vi "test Connector Pane.vi"(8 "error in (no error)":errorcluster, 11 "TestCase in":refnum<class "Embedded Data Logger Unit Tests.lvclass">) -> (0 "error out":errorcluster, 3 "TestCase out":refnum<class "Embedded Data Logger Unit Tests.lvclass">)   [LabVIEW 2027, in "Embedded Data Logger Unit Tests.lvclass"]
uses:
  Embedded Data Logger Unit Tests.lvclass
  C:/Program Files/National Instruments/LabVIEW 2027/vi.lib/addons/_JKI Toolkits/VI Tester/TestCase.llb/TestCase.lvclass
  <vilib>/addons/_JKI Toolkits/VI Tester/TestCase.llb/TestCase.lvclass
  <vilib>/NI/VeriStand Custom Device Testing Tools/VeriStandTestUtilities/VeriStandTestUtilities.lvlib
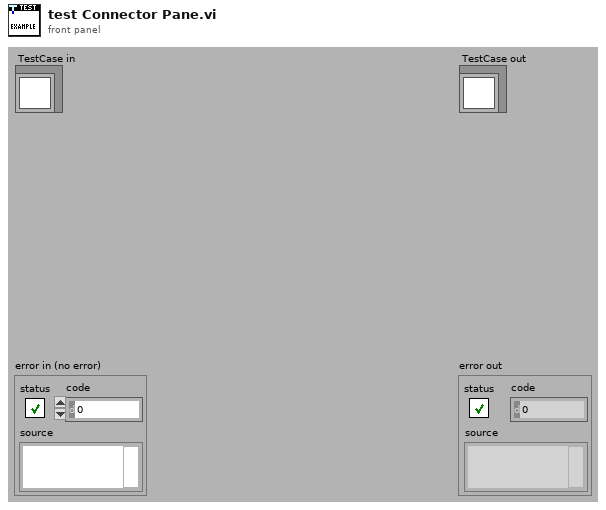
[diagram p1: front panel]
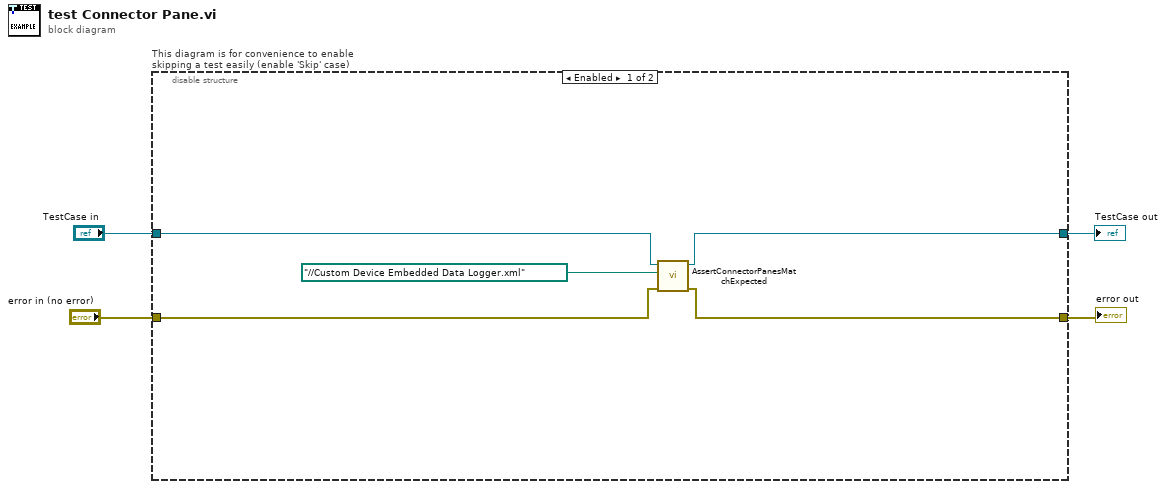
[diagram p0: block diagram]
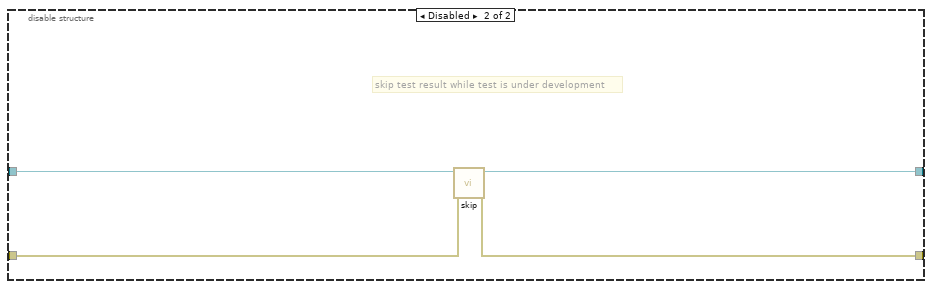
[diagram p2: hidden frame]
diagram:
  n1 = disable-structure "This diagram is for convenience to enable skipping a test easily (enable 'Skip' case)" shown="Enabled" {
    disable-tunnel: "TestCase in" -> [w9 w13]
    disable-tunnel: [w8 w11] -> w1
    disable-tunnel: [w7 w12] -> w3
    disable-tunnel: "error in (no error)" -> [w6 w10]
    frame Enabled {
      n2 = call <vilib>:"AssertConnectorPanesMatchExpected.vi"("error in (no error)"=w6, "custom device xml path"=path "../../Custom Device Embedded Data Logger.xml", "TestCase in"=w9) -> ("error out"=w7:errorcluster, "TestCase out"=w8:refnum<class "Embedded Data Logger Unit Tests.lvclass">)  [unwired: 7 in]
    }
    frame Disabled {
      # "skip test result while test is under development"
      n3 = call <vilib>:"skip.vi"("error in (no error)"=w10, "TestCase in"=w13) -> ("error out"=w12:errorcluster, "TestCase out"=w11:refnum<class "Embedded Data Logger Unit Tests.lvclass">)  [unwired: 8 in]
    }
  }
  "error out" <- w3
  "TestCase out" <- w1
